vi "Entrenamiento Fuerza 2.vi"(8 "error in (no error)":errorcluster) -> (0 "error out":errorcluster, 3 "Message":string)   [LabVIEW 2014]
panel:
  out "Horizontal Graduated Bar":i16(slide) scale=0.0..100.0
  in  "Remove Button":bool
  in  "Add Button":bool
  out "Opcional %":string="0%"
  in  "Opcional Bool":bool
  out "Biceps %":string="0%"
  in  "Biceps Bool":bool
  out "Pectorales %":string="0%"
  in  "Pectorales Bool":bool
  out "Trapecio %":string="0%"
  in  "Trapecio Bool":bool
  out "Dorsales %":string="0%"
  in  "Dorsales Bool":bool
  out "Lumbares %":string="0%"
  in  "Lumbares Bool":bool
  out "Abdomen %":string="0%"
  in  "Abdomen Bool":bool
  out "Gluteos %":string="0%"
  in  "Gluteos Bool":bool
  out "Isquiotibiales %":string="0%"
  in  "Isquiotibiales Bool":bool
  in  "Stop":bool
  out "Cuadríceps %":string="0%"
  in  "Cuadriceps Bool":bool
  out "date/time string":string="22/08/2015 01:25:29 a. m."
  # "Entrenamiento de Fuerza"
  # "Presentación"
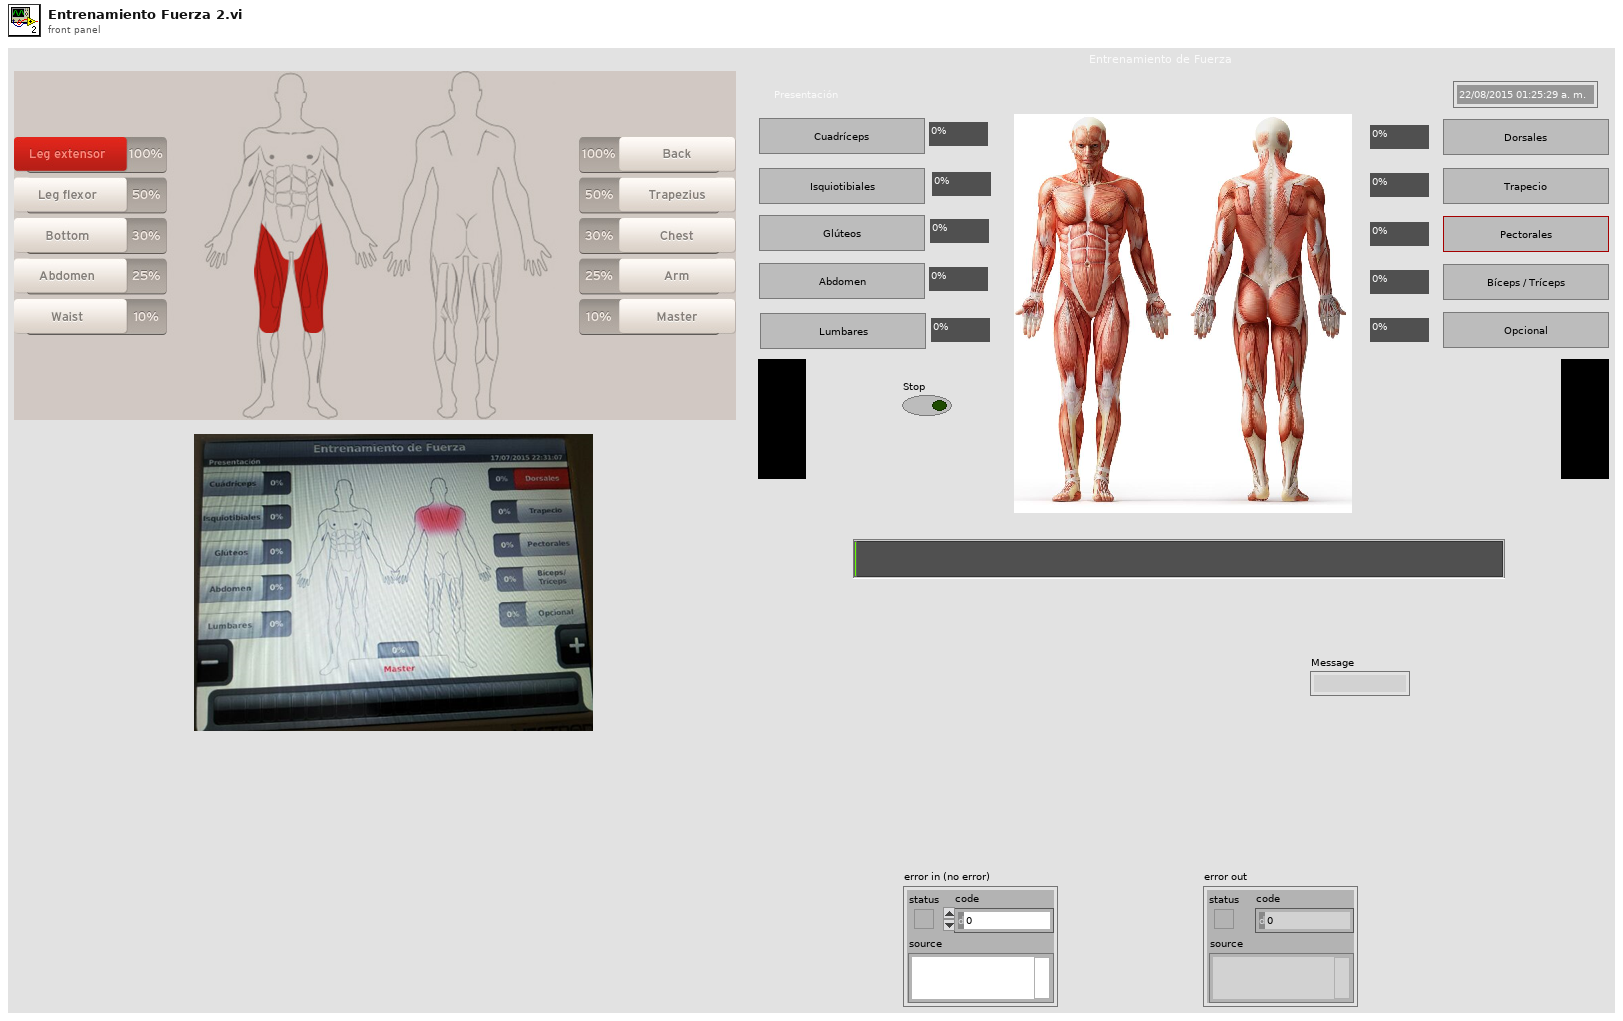
[diagram p1: front panel]
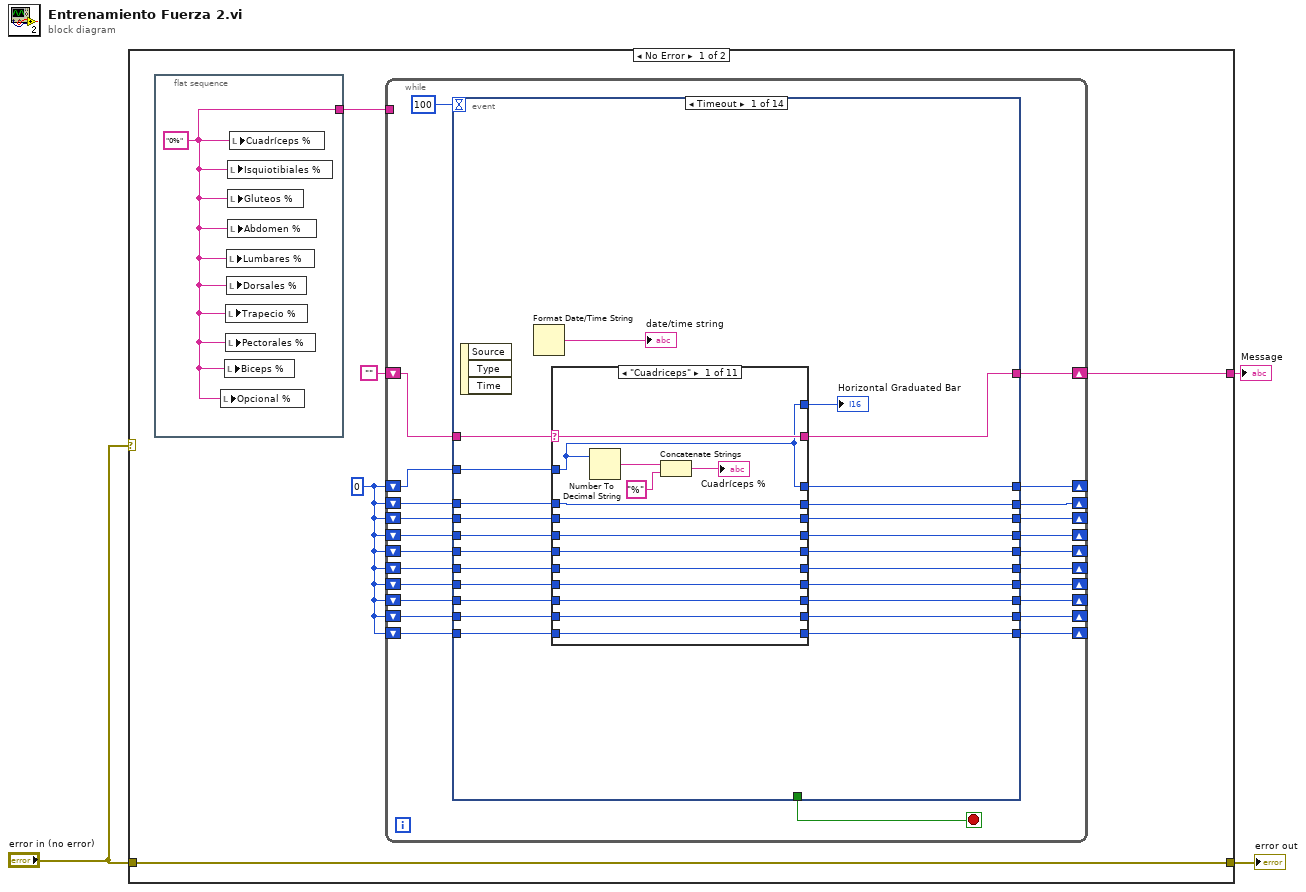
[diagram p0: block diagram]
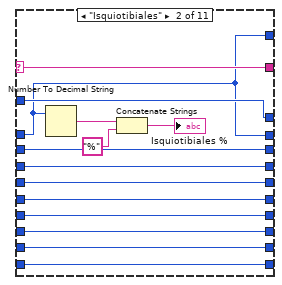
[diagram p2: hidden frame]
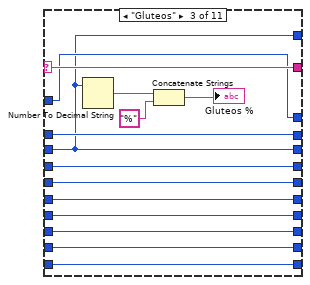
[diagram p3: hidden frame]
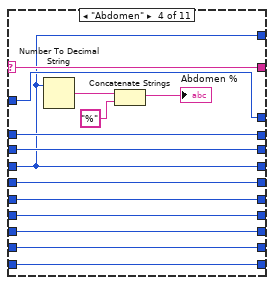
[diagram p4: hidden frame]
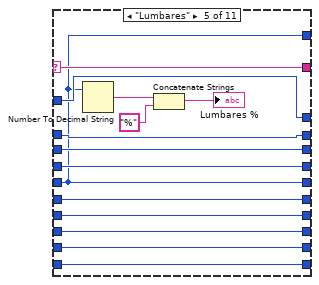
[diagram p5: hidden frame]
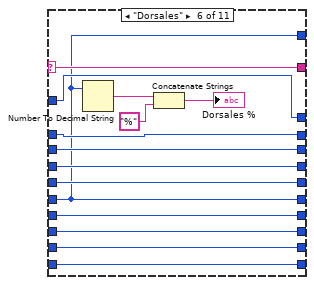
[diagram p6: hidden frame]
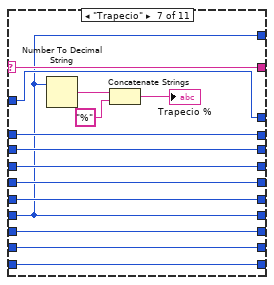
[diagram p7: hidden frame]
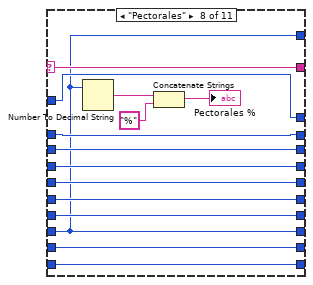
[diagram p8: hidden frame]
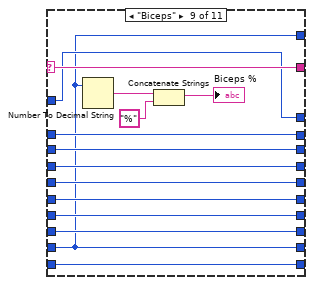
[diagram p9: hidden frame]
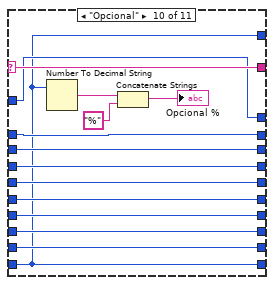
[diagram p10: hidden frame]
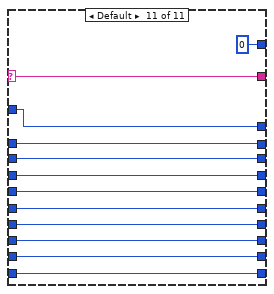
[diagram p11: hidden frame]
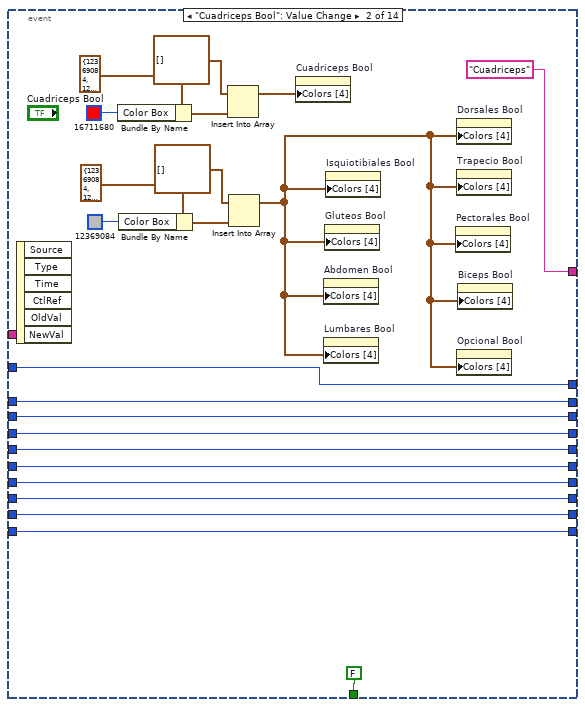
[diagram p12: hidden frame]
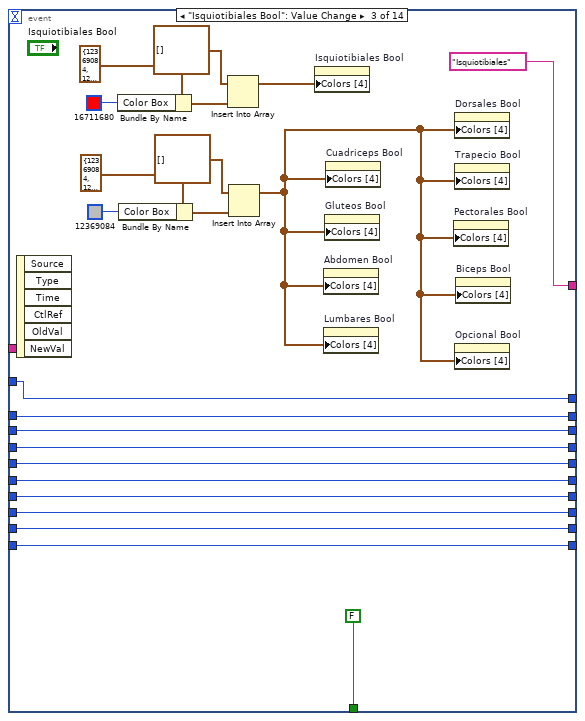
[diagram p13: hidden frame]
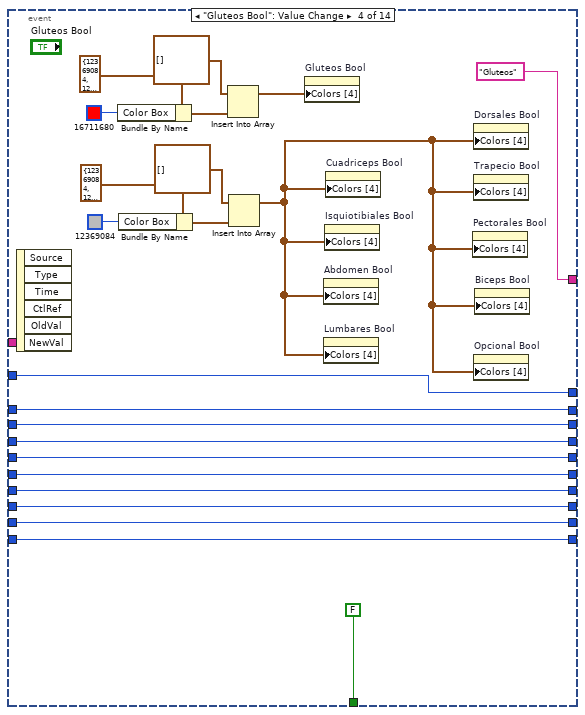
[diagram p14: hidden frame]
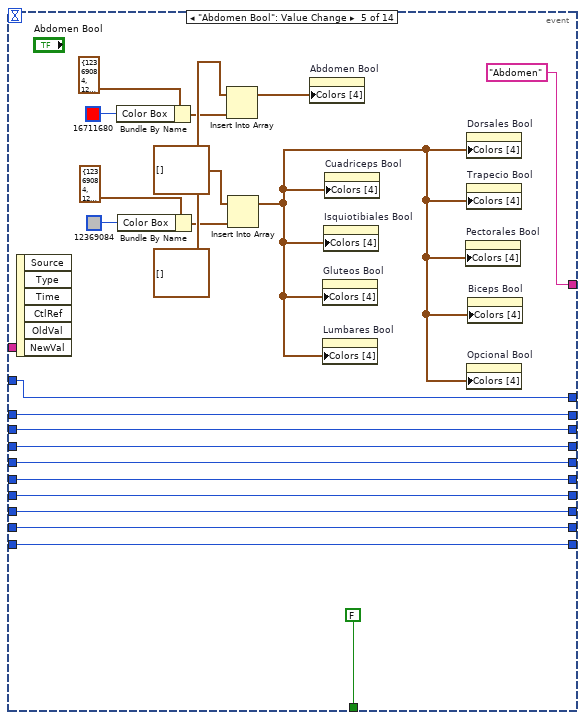
[diagram p15: hidden frame]
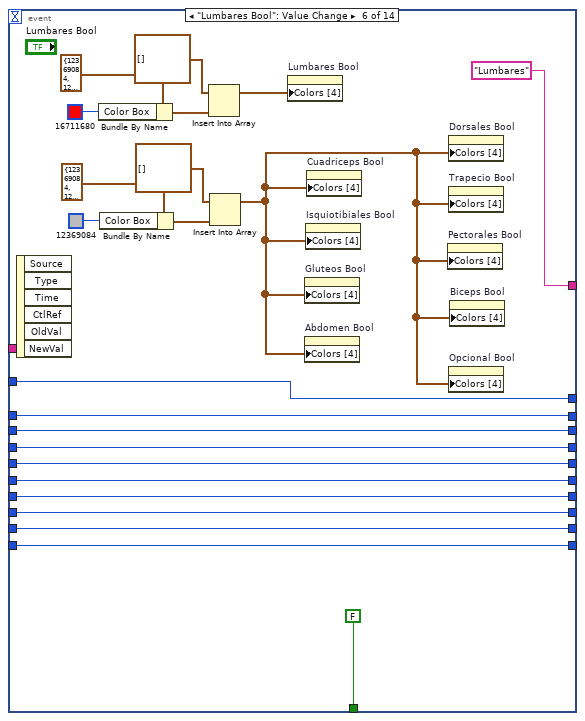
[diagram p16: hidden frame]
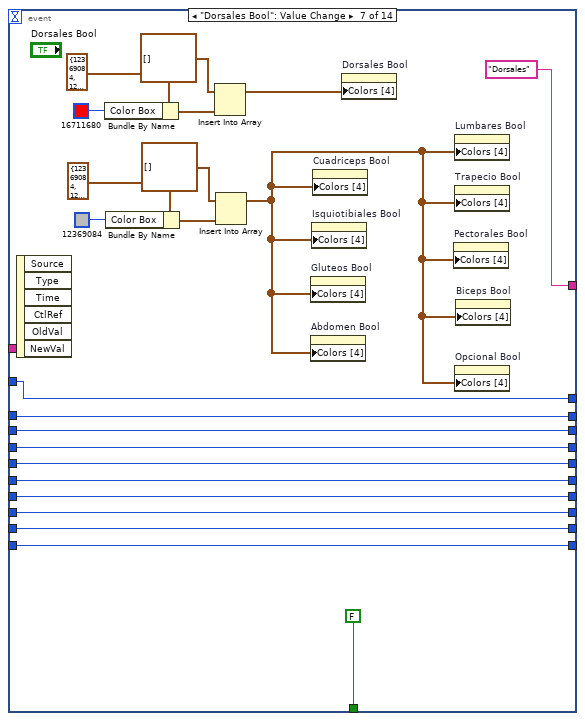
[diagram p17: hidden frame]
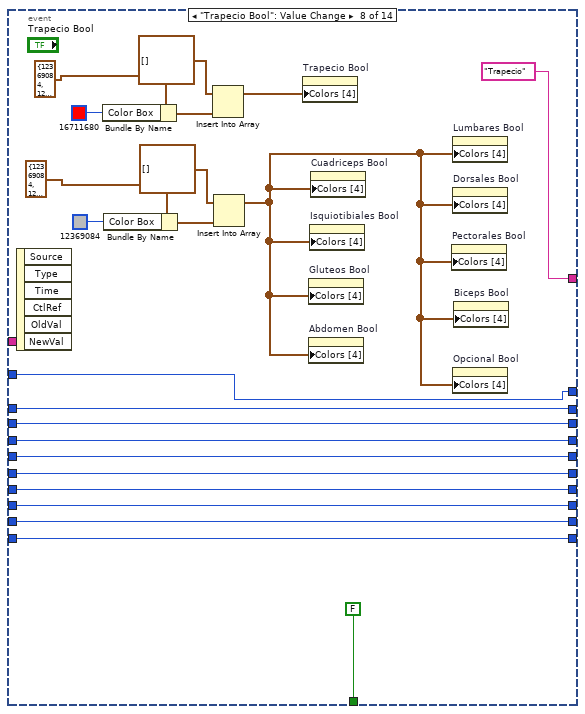
[diagram p18: hidden frame]
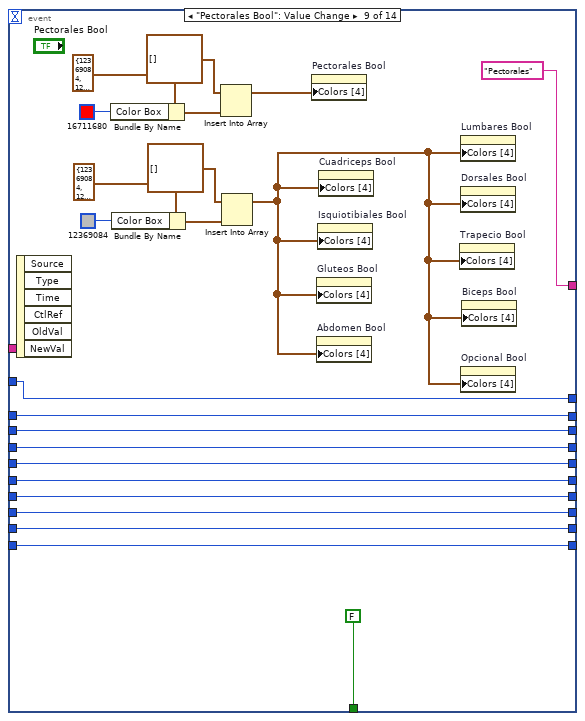
[diagram p19: hidden frame]
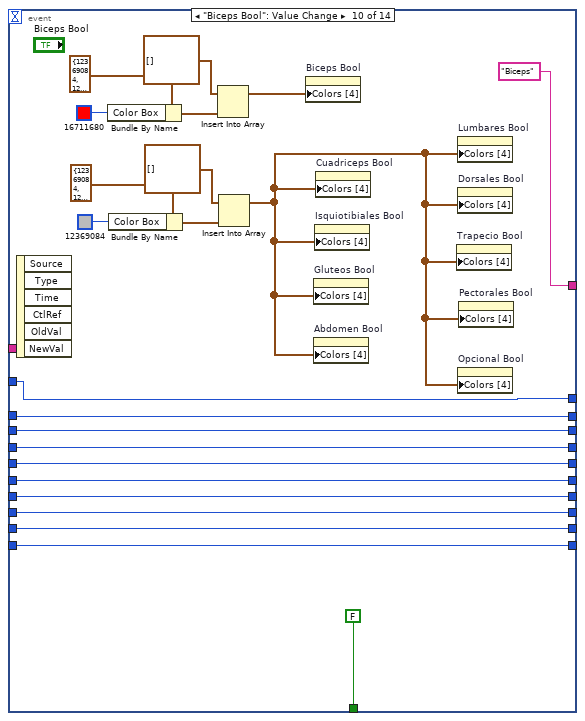
[diagram p20: hidden frame]
diagram:
  n1 = case shown="No Error" "error in (no error)" {
    tunnel: "error in (no error)" -> [w8 w815]
    tunnel: [w8 w815] -> w2
    tunnel: [w7 "Error" ("Message")] -> w1
    frame No Error {
      w5 = 0
      n2 = flat-sequence {
        tunnel: [w9] -> w4
        frame #0 {
          w9 = "0%" ("Cuadríceps %")
          n3 = local write "Opcional %"(w9) -> ()
          n4 = local write "Biceps %"(w9) -> ()
          n5 = local write "Trapecio %"(w9) -> ()
          n6 = local write "Pectorales %"(w9) -> ()
          n7 = local write "Lumbares %"(w9) -> ()
          n8 = local write "Dorsales %"(w9) -> ()
          n9 = local write "Isquiotibiales %"(w9) -> ()
          n10 = local write "Gluteos %"(w9) -> ()
          n11 = local write "Abdomen %"(w9) -> ()
          n12 = local write "Cuadríceps %"(w9) -> ()
        }
      }
      n13 = while {
        shift-right: [w31] -> w7
        shift-left: "" ("Message") -> [w30]
        shift-right: [w10] -> _
        shift-left: w5 -> [w29]
        shift-right: [w11] -> _
        shift-left: w5 -> [w28]
        shift-right: [w12] -> _
        shift-left: w5 -> [w27]
        shift-right: [w13] -> _
        shift-left: w5 -> [w26]
        shift-right: [w14] -> _
        shift-left: w5 -> [w25]
        shift-right: [w15] -> _
        shift-left: w5 -> [w24]
        shift-right: [w16] -> _
        shift-left: w5 -> [w23]
        shift-right: [w17] -> _
        shift-left: w5 -> [w22]
        shift-right: [w18] -> _
        shift-left: w5 -> [w21]
        shift-right: [w19] -> _
        shift-left: w5 -> [w20]
        tunnel: w4 -> [_]
        stop <- w33 stop-if-true
        n14 = event shown="[0] Timeout" {
          selector: _ -> [_ _ _ _ _ _ _ _ _ _ _ _ _ _]
          dyn-events: _ -> [_ _ _ _ _ _ _ _ _ _ _ _ _ _]
          timeout: 100 -> [_ _ _ _ _ _ _ _ _ _ _ _ _ _]
          tunnel: [_ FALSE FALSE FALSE FALSE FALSE FALSE FALSE FALSE FALSE FALSE _ _ "Stop"] -> w33
          tunnel: [w55 "Cuadriceps" ("Message") "Isquiotibiales" ("Message") "Gluteos" ("Message") "Abdomen" ("Message") "Lumbares" ("Message") "Dorsales" ("Message") "Trapecio" ("Message") "Pectorales" ("Message") "Biceps" ("Message") "Opcional" ("Message") w450 w651 w812] -> w31
          tunnel: w30 -> [w56 _ _ _ _ _ _ _ _ _ _ w450 w651 w812]
          tunnel: w29 -> [w54 w210 w241 w254 w276 w298 w329 w351 w364 w395 w417 w449 w650 w802]
          tunnel: w28 -> [w53 w211 w240 w255 w277 w299 w328 w350 w373 w394 w416 w440 w641 w803]
          tunnel: w27 -> [w52 w212 w239 w256 w278 w300 w327 w349 w372 w393 w415 w441 w642 w804]
          tunnel: w26 -> [w51 w213 w238 w257 w279 w301 w326 w348 w371 w392 w414 w442 w643 w805]
          tunnel: w25 -> [w50 w214 w237 w258 w280 w302 w325 w347 w370 w391 w413 w443 w644 w806]
          tunnel: w24 -> [w49 w215 w236 w259 w281 w303 w324 w346 w369 w390 w412 w444 w645 w807]
          tunnel: w23 -> [w48 w216 w235 w260 w282 w304 w323 w345 w368 w389 w411 w445 w646 w808]
          tunnel: w22 -> [w35 w217 w234 w261 w283 w305 w322 w344 w367 w388 w410 w446 w647 w809]
          tunnel: w21 -> [w47 w218 w233 w262 w284 w306 w321 w343 w366 w387 w409 w447 w648 w810]
          tunnel: w20 -> [w46 w219 w232 w263 w285 w307 w320 w342 w365 w386 w408 w448 w649 w811]
          tunnel: [w45 w219 w232 w263 w285 w307 w320 w342 w365 w386 w408 w431 w632 w811] -> w19
          tunnel: [w44 w218 w233 w262 w284 w306 w321 w343 w366 w387 w409 w432 w633 w810] -> w18
          tunnel: [w43 w217 w234 w261 w283 w305 w322 w344 w367 w388 w410 w433 w634 w809] -> w17
          tunnel: [w42 w216 w235 w260 w282 w304 w323 w345 w368 w389 w411 w434 w635 w808] -> w16
          tunnel: [w41 w215 w236 w259 w281 w303 w324 w346 w369 w390 w412 w435 w636 w807] -> w15
          tunnel: [w40 w214 w237 w258 w280 w302 w325 w347 w370 w391 w413 w436 w637 w806] -> w14
          tunnel: [w39 w213 w238 w257 w279 w301 w326 w348 w371 w392 w414 w437 w638 w805] -> w13
          tunnel: [w38 w212 w239 w256 w278 w300 w327 w349 w372 w393 w415 w438 w639 w804] -> w12
          tunnel: [w37 w211 w240 w255 w277 w299 w328 w350 w373 w394 w416 w439 w640 w803] -> w11
          tunnel: [w36 w210 w241 w254 w276 w298 w329 w351 w364 w395 w417 w430 w631 w802] -> w10
          event Timeout {
            n15 = event-data() -> ()  [unwired: 1 in, 3 out]
            n16 = Format Date/Time String() -> (date/time string=→"date/time string":string)  [unwired: 3 in]
            n17 = case shown="\"Cuadriceps\"" w56 {
              selector: w56 -> [w71 w85 w99 w113 w127 w141 w155 w169 w183 w197 w209]
              tunnel: [w71 w85 w99 w113 w127 w141 w155 w169 w183 w197 w209] -> w55
              tunnel: w54 -> [w58 w73 w87 w101 w115 w129 w143 w157 w171 w186 w208]
              tunnel: w53 -> [w59 w72 w88 w102 w116 w130 w144 w158 w172 w185 w207]
              tunnel: w52 -> [w60 w74 w86 w103 w117 w135 w145 w159 w173 w187 w206]
              tunnel: w51 -> [w61 w75 w89 w100 w118 w136 w146 w165 w174 w188 w205]
              tunnel: w50 -> [w62 w76 w90 w104 w114 w137 w147 w164 w175 w189 w204]
              tunnel: w49 -> [w63 w77 w91 w105 w123 w128 w148 w163 w176 w190 w203]
              tunnel: w48 -> [w64 w78 w92 w106 w122 w134 w142 w162 w177 w191 w202]
              tunnel: w47 -> [w66 w80 w94 w108 w120 w132 w151 w161 w170 w193 w200]
              tunnel: w46 -> [w67 w81 w95 w109 w119 w131 w149 w160 w179 w184 w199]
              tunnel: [w67 w81 w95 w109 w119 w131 w149 w160 w179 w184 w199] -> w45
              tunnel: [w66 w80 w94 w108 w120 w132 w151 w161 w170 w193 w200] -> w44
              tunnel: [w65 w79 w93 w107 w121 w133 w150 w156 w178 w192 w201] -> w43
              tunnel: [w64 w78 w92 w106 w122 w134 w142 w162 w177 w191 w202] -> w42
              tunnel: [w63 w77 w91 w105 w123 w128 w148 w163 w176 w190 w203] -> w41
              tunnel: [w62 w76 w90 w104 w114 w137 w147 w164 w175 w189 w204] -> w40
              tunnel: [w61 w75 w89 w100 w118 w136 w146 w165 w174 w188 w205] -> w39
              tunnel: [w60 w74 w86 w103 w117 w135 w145 w159 w173 w187 w206] -> w38
              tunnel: [w59 w72 w88 w102 w116 w130 w144 w158 w172 w185 w207] -> w37
              tunnel: [w58 w73 w87 w101 w115 w129 w143 w157 w171 w186 w208] -> w36
              tunnel: w35 -> [w65 w79 w93 w107 w121 w133 w150 w156 w178 w192 w201]
              tunnel: [w58 w72 w86 w100 w114 w128 w142 w156 w170 w184 0] -> w34
              frame "Cuadriceps" {
                n18 = Number To Decimal String(number=w58) -> (decimal integer string=w70:string)  [unwired: 1 in]
                n19 = Concatenate Strings(w70, "%" ("string")) -> (→"Cuadríceps %":string)
              }
              frame "Isquiotibiales" {
                n20 = Number To Decimal String(number=w72) -> (decimal integer string=w84:string)  [unwired: 1 in]
                n21 = Concatenate Strings(w84, "%" ("string")) -> (→"Isquiotibiales %":string)
              }
              frame "Gluteos" {
                n22 = Number To Decimal String(number=w86) -> (decimal integer string=w98:string)  [unwired: 1 in]
                n23 = Concatenate Strings(w98, "%" ("string")) -> (→"Gluteos %":string)
              }
              frame "Abdomen" {
                n24 = Number To Decimal String(number=w100) -> (decimal integer string=w112:string)  [unwired: 1 in]
                n25 = Concatenate Strings(w112, "%" ("string")) -> (→"Abdomen %":string)
              }
              frame "Lumbares" {
                n26 = Number To Decimal String(number=w114) -> (decimal integer string=w126:string)  [unwired: 1 in]
                n27 = Concatenate Strings(w126, "%" ("string")) -> (→"Lumbares %":string)
              }
              frame "Dorsales" {
                n28 = Number To Decimal String(number=w128) -> (decimal integer string=w140:string)  [unwired: 1 in]
                n29 = Concatenate Strings(w140, "%" ("string")) -> (→"Dorsales %":string)
              }
              frame "Trapecio" {
                n30 = Number To Decimal String(number=w142) -> (decimal integer string=w154:string)  [unwired: 1 in]
                n31 = Concatenate Strings(w154, "%" ("string")) -> (→"Trapecio %":string)
              }
              frame "Pectorales" {
                n32 = Number To Decimal String(number=w156) -> (decimal integer string=w168:string)  [unwired: 1 in]
                n33 = Concatenate Strings(w168, "%" ("string")) -> (→"Pectorales %":string)
              }
              frame "Biceps" {
                n34 = Number To Decimal String(number=w170) -> (decimal integer string=w182:string)  [unwired: 1 in]
                n35 = Concatenate Strings(w182, "%" ("string")) -> (→"Biceps %":string)
              }
              frame "Opcional" {
                n36 = Number To Decimal String(number=w184) -> (decimal integer string=w196:string)  [unwired: 1 in]
                n37 = Concatenate Strings(w196, "%" ("string")) -> (→"Opcional %":string)
              }
              frame Default {
              }
            }
            "Horizontal Graduated Bar" <- w34
          }
          event "Cuadriceps Bool": Value Change {
            n38 = event-data() -> ()  [unwired: 1 in, 6 out]
            n39 = Bundle By Name(cluster=cluster{"Color Box":u32, "Color Box 2":u32} {"Color Box"=12369084, "Color Box 2"=12369084}, "Color Box"=u32 16711680 ("Color Box 2")) -> (w228:cluster{"Color Box":u32, "Color Box 2":u32})
            n40 = Bundle By Name(cluster=cluster{"Color Box":u32, "Color Box 2":u32} {"Color Box"=12369084, "Color Box 2"=12369084}, "Color Box"=u32 12369084 ("Color Box 2")) -> (w223:cluster{"Color Box":u32, "Color Box 2":u32})
            n41 = Insert Into Array(array=cluster{u32, u32}[] [] ("Colors [4]"), new element=w228) -> (w227:cluster{u32, u32}[])  [unwired: 1 in]
            n42 = Insert Into Array(array=cluster{u32, u32}[] [] ("Colors [4]"), new element=w223) -> (w221:cluster{u32, u32}[])  [unwired: 1 in]
            n43 = property on="Cuadriceps Bool" class="Bool"("Colors [4]"=w227) -> ()  [unwired: 2 in, 2 out]
            n44 = property on="Abdomen Bool" class="Bool"("Colors [4]"=w221) -> ()  [unwired: 2 in, 2 out]
            n45 = property on="Lumbares Bool" class="Bool"("Colors [4]"=w221) -> ()  [unwired: 2 in, 2 out]
            n46 = property on="Gluteos Bool" class="Bool"("Colors [4]"=w221) -> ()  [unwired: 2 in, 2 out]
            n47 = property on="Isquiotibiales Bool" class="Bool"("Colors [4]"=w221) -> ()  [unwired: 2 in, 2 out]
            n48 = property on="Pectorales Bool" class="Bool"("Colors [4]"=w221) -> ()  [unwired: 2 in, 2 out]
            n49 = property on="Dorsales Bool" class="Bool"("Colors [4]"=w221) -> ()  [unwired: 2 in, 2 out]
            n50 = property on="Trapecio Bool" class="Bool"("Colors [4]"=w221) -> ()  [unwired: 2 in, 2 out]
            n51 = property on="Opcional Bool" class="Bool"("Colors [4]"=w221) -> ()  [unwired: 2 in, 2 out]
            n52 = property on="Biceps Bool" class="Bool"("Colors [4]"=w221) -> ()  [unwired: 2 in, 2 out]
          }
          event "Isquiotibiales Bool": Value Change {
            n53 = event-data() -> ()  [unwired: 1 in, 6 out]
            n54 = Bundle By Name(cluster=cluster{"Color Box":u32, "Color Box 2":u32} {"Color Box"=12369084, "Color Box 2"=12369084}, "Color Box"=u32 16711680 ("Color Box 2")) -> (w249:cluster{"Color Box":u32, "Color Box 2":u32})
            n55 = Bundle By Name(cluster=cluster{"Color Box":u32, "Color Box 2":u32} {"Color Box"=12369084, "Color Box 2"=12369084}, "Color Box"=u32 12369084 ("Color Box 2")) -> (w245:cluster{"Color Box":u32, "Color Box 2":u32})
            n56 = Insert Into Array(array=cluster{u32, u32}[] [] ("Colors [4]"), new element=w249) -> (w243:cluster{u32, u32}[])  [unwired: 1 in]
            n57 = Insert Into Array(array=cluster{u32, u32}[] [] ("Colors [4]"), new element=w245) -> (w242:cluster{u32, u32}[])  [unwired: 1 in]
            n58 = property on="Isquiotibiales Bool" class="Bool"("Colors [4]"=w243) -> ()  [unwired: 2 in, 2 out]
            n59 = property on="Abdomen Bool" class="Bool"("Colors [4]"=w242) -> ()  [unwired: 2 in, 2 out]
            n60 = property on="Lumbares Bool" class="Bool"("Colors [4]"=w242) -> ()  [unwired: 2 in, 2 out]
            n61 = property on="Gluteos Bool" class="Bool"("Colors [4]"=w242) -> ()  [unwired: 2 in, 2 out]
            n62 = property on="Cuadriceps Bool" class="Bool"("Colors [4]"=w242) -> ()  [unwired: 2 in, 2 out]
            n63 = property on="Pectorales Bool" class="Bool"("Colors [4]"=w242) -> ()  [unwired: 2 in, 2 out]
            n64 = property on="Dorsales Bool" class="Bool"("Colors [4]"=w242) -> ()  [unwired: 2 in, 2 out]
            n65 = property on="Trapecio Bool" class="Bool"("Colors [4]"=w242) -> ()  [unwired: 2 in, 2 out]
            n66 = property on="Opcional Bool" class="Bool"("Colors [4]"=w242) -> ()  [unwired: 2 in, 2 out]
            n67 = property on="Biceps Bool" class="Bool"("Colors [4]"=w242) -> ()  [unwired: 2 in, 2 out]
          }
          event "Gluteos Bool": Value Change {
            n68 = event-data() -> ()  [unwired: 1 in, 6 out]
            n69 = Bundle By Name(cluster=cluster{"Color Box":u32, "Color Box 2":u32} {"Color Box"=12369084, "Color Box 2"=12369084}, "Color Box"=u32 16711680 ("Color Box 2")) -> (w271:cluster{"Color Box":u32, "Color Box 2":u32})
            n70 = Bundle By Name(cluster=cluster{"Color Box":u32, "Color Box 2":u32} {"Color Box"=12369084, "Color Box 2"=12369084}, "Color Box"=u32 12369084 ("Color Box 2")) -> (w267:cluster{"Color Box":u32, "Color Box 2":u32})
            n71 = Insert Into Array(array=cluster{u32, u32}[] [] ("Colors [4]"), new element=w271) -> (w265:cluster{u32, u32}[])  [unwired: 1 in]
            n72 = Insert Into Array(array=cluster{u32, u32}[] [] ("Colors [4]"), new element=w267) -> (w264:cluster{u32, u32}[])  [unwired: 1 in]
            n73 = property on="Gluteos Bool" class="Bool"("Colors [4]"=w265) -> ()  [unwired: 2 in, 2 out]
            n74 = property on="Abdomen Bool" class="Bool"("Colors [4]"=w264) -> ()  [unwired: 2 in, 2 out]
            n75 = property on="Lumbares Bool" class="Bool"("Colors [4]"=w264) -> ()  [unwired: 2 in, 2 out]
            n76 = property on="Isquiotibiales Bool" class="Bool"("Colors [4]"=w264) -> ()  [unwired: 2 in, 2 out]
            n77 = property on="Cuadriceps Bool" class="Bool"("Colors [4]"=w264) -> ()  [unwired: 2 in, 2 out]
            n78 = property on="Pectorales Bool" class="Bool"("Colors [4]"=w264) -> ()  [unwired: 2 in, 2 out]
            n79 = property on="Dorsales Bool" class="Bool"("Colors [4]"=w264) -> ()  [unwired: 2 in, 2 out]
            n80 = property on="Trapecio Bool" class="Bool"("Colors [4]"=w264) -> ()  [unwired: 2 in, 2 out]
            n81 = property on="Opcional Bool" class="Bool"("Colors [4]"=w264) -> ()  [unwired: 2 in, 2 out]
            n82 = property on="Biceps Bool" class="Bool"("Colors [4]"=w264) -> ()  [unwired: 2 in, 2 out]
          }
          event "Abdomen Bool": Value Change {
            n83 = event-data() -> ()  [unwired: 1 in, 6 out]
            n84 = Bundle By Name(cluster=cluster{"Color Box":u32, "Color Box 2":u32} {"Color Box"=12369084, "Color Box 2"=12369084}, "Color Box"=u32 16711680 ("Color Box 2")) -> (w293:cluster{"Color Box":u32, "Color Box 2":u32})
            n85 = Bundle By Name(cluster=cluster{"Color Box":u32, "Color Box 2":u32} {"Color Box"=12369084, "Color Box 2"=12369084}, "Color Box"=u32 12369084 ("Color Box 2")) -> (w289:cluster{"Color Box":u32, "Color Box 2":u32})
            n86 = Insert Into Array(array=cluster{u32, u32}[] [] ("Colors [4]"), new element=w293) -> (w287:cluster{u32, u32}[])  [unwired: 1 in]
            n87 = Insert Into Array(array=cluster{u32, u32}[] [] ("Colors [4]"), new element=w289) -> (w286:cluster{u32, u32}[])  [unwired: 1 in]
            n88 = property on="Abdomen Bool" class="Bool"("Colors [4]"=w287) -> ()  [unwired: 2 in, 2 out]
            n89 = property on="Gluteos Bool" class="Bool"("Colors [4]"=w286) -> ()  [unwired: 2 in, 2 out]
            n90 = property on="Lumbares Bool" class="Bool"("Colors [4]"=w286) -> ()  [unwired: 2 in, 2 out]
            n91 = property on="Isquiotibiales Bool" class="Bool"("Colors [4]"=w286) -> ()  [unwired: 2 in, 2 out]
            n92 = property on="Cuadriceps Bool" class="Bool"("Colors [4]"=w286) -> ()  [unwired: 2 in, 2 out]
            n93 = property on="Pectorales Bool" class="Bool"("Colors [4]"=w286) -> ()  [unwired: 2 in, 2 out]
            n94 = property on="Dorsales Bool" class="Bool"("Colors [4]"=w286) -> ()  [unwired: 2 in, 2 out]
            n95 = property on="Trapecio Bool" class="Bool"("Colors [4]"=w286) -> ()  [unwired: 2 in, 2 out]
            n96 = property on="Opcional Bool" class="Bool"("Colors [4]"=w286) -> ()  [unwired: 2 in, 2 out]
            n97 = property on="Biceps Bool" class="Bool"("Colors [4]"=w286) -> ()  [unwired: 2 in, 2 out]
          }
          event "Lumbares Bool": Value Change {
            n98 = event-data() -> ()  [unwired: 1 in, 6 out]
            n99 = Bundle By Name(cluster=cluster{"Color Box":u32, "Color Box 2":u32} {"Color Box"=12369084, "Color Box 2"=12369084}, "Color Box"=u32 16711680 ("Color Box 2")) -> (w315:cluster{"Color Box":u32, "Color Box 2":u32})
            n100 = Bundle By Name(cluster=cluster{"Color Box":u32, "Color Box 2":u32} {"Color Box"=12369084, "Color Box 2"=12369084}, "Color Box"=u32 12369084 ("Color Box 2")) -> (w311:cluster{"Color Box":u32, "Color Box 2":u32})
            n101 = Insert Into Array(array=cluster{u32, u32}[] [] ("Colors [4]"), new element=w315) -> (w309:cluster{u32, u32}[])  [unwired: 1 in]
            n102 = Insert Into Array(array=cluster{u32, u32}[] [] ("Colors [4]"), new element=w311) -> (w308:cluster{u32, u32}[])  [unwired: 1 in]
            n103 = property on="Lumbares Bool" class="Bool"("Colors [4]"=w309) -> ()  [unwired: 2 in, 2 out]
            n104 = property on="Gluteos Bool" class="Bool"("Colors [4]"=w308) -> ()  [unwired: 2 in, 2 out]
            n105 = property on="Abdomen Bool" class="Bool"("Colors [4]"=w308) -> ()  [unwired: 2 in, 2 out]
            n106 = property on="Isquiotibiales Bool" class="Bool"("Colors [4]"=w308) -> ()  [unwired: 2 in, 2 out]
            n107 = property on="Cuadriceps Bool" class="Bool"("Colors [4]"=w308) -> ()  [unwired: 2 in, 2 out]
            n108 = property on="Pectorales Bool" class="Bool"("Colors [4]"=w308) -> ()  [unwired: 2 in, 2 out]
            n109 = property on="Dorsales Bool" class="Bool"("Colors [4]"=w308) -> ()  [unwired: 2 in, 2 out]
            n110 = property on="Trapecio Bool" class="Bool"("Colors [4]"=w308) -> ()  [unwired: 2 in, 2 out]
            n111 = property on="Opcional Bool" class="Bool"("Colors [4]"=w308) -> ()  [unwired: 2 in, 2 out]
            n112 = property on="Biceps Bool" class="Bool"("Colors [4]"=w308) -> ()  [unwired: 2 in, 2 out]
          }
          event "Dorsales Bool": Value Change {
            n113 = event-data() -> ()  [unwired: 1 in, 6 out]
            n114 = Bundle By Name(cluster=cluster{"Color Box":u32, "Color Box 2":u32} {"Color Box"=12369084, "Color Box 2"=12369084}, "Color Box"=u32 16711680 ("Color Box 2")) -> (w337:cluster{"Color Box":u32, "Color Box 2":u32})
            n115 = Bundle By Name(cluster=cluster{"Color Box":u32, "Color Box 2":u32} {"Color Box"=12369084, "Color Box 2"=12369084}, "Color Box"=u32 12369084 ("Color Box 2")) -> (w333:cluster{"Color Box":u32, "Color Box 2":u32})
            n116 = Insert Into Array(array=cluster{u32, u32}[] [] ("Colors [4]"), new element=w337) -> (w330:cluster{u32, u32}[])  [unwired: 1 in]
            n117 = Insert Into Array(array=cluster{u32, u32}[] [] ("Colors [4]"), new element=w333) -> (w331:cluster{u32, u32}[])  [unwired: 1 in]
            n118 = property on="Gluteos Bool" class="Bool"("Colors [4]"=w331) -> ()  [unwired: 2 in, 2 out]
            n119 = property on="Abdomen Bool" class="Bool"("Colors [4]"=w331) -> ()  [unwired: 2 in, 2 out]
            n120 = property on="Isquiotibiales Bool" class="Bool"("Colors [4]"=w331) -> ()  [unwired: 2 in, 2 out]
            n121 = property on="Cuadriceps Bool" class="Bool"("Colors [4]"=w331) -> ()  [unwired: 2 in, 2 out]
            n122 = property on="Dorsales Bool" class="Bool"("Colors [4]"=w330) -> ()  [unwired: 2 in, 2 out]
            n123 = property on="Pectorales Bool" class="Bool"("Colors [4]"=w331) -> ()  [unwired: 2 in, 2 out]
            n124 = property on="Lumbares Bool" class="Bool"("Colors [4]"=w331) -> ()  [unwired: 2 in, 2 out]
            n125 = property on="Trapecio Bool" class="Bool"("Colors [4]"=w331) -> ()  [unwired: 2 in, 2 out]
            n126 = property on="Opcional Bool" class="Bool"("Colors [4]"=w331) -> ()  [unwired: 2 in, 2 out]
            n127 = property on="Biceps Bool" class="Bool"("Colors [4]"=w331) -> ()  [unwired: 2 in, 2 out]
          }
          event "Trapecio Bool": Value Change {
            n128 = event-data() -> ()  [unwired: 1 in, 6 out]
            n129 = Bundle By Name(cluster=cluster{"Color Box":u32, "Color Box 2":u32} {"Color Box"=12369084, "Color Box 2"=12369084}, "Color Box"=u32 16711680 ("Color Box 2")) -> (w359:cluster{"Color Box":u32, "Color Box 2":u32})
            n130 = Bundle By Name(cluster=cluster{"Color Box":u32, "Color Box 2":u32} {"Color Box"=12369084, "Color Box 2"=12369084}, "Color Box"=u32 12369084 ("Color Box 2")) -> (w355:cluster{"Color Box":u32, "Color Box 2":u32})
            n131 = Insert Into Array(array=cluster{u32, u32}[] [] ("Colors [4]"), new element=w359) -> (w352:cluster{u32, u32}[])  [unwired: 1 in]
            n132 = Insert Into Array(array=cluster{u32, u32}[] [] ("Colors [4]"), new element=w355) -> (w353:cluster{u32, u32}[])  [unwired: 1 in]
            n133 = property on="Trapecio Bool" class="Bool"("Colors [4]"=w352) -> ()  [unwired: 2 in, 2 out]
            n134 = property on="Gluteos Bool" class="Bool"("Colors [4]"=w353) -> ()  [unwired: 2 in, 2 out]
            n135 = property on="Abdomen Bool" class="Bool"("Colors [4]"=w353) -> ()  [unwired: 2 in, 2 out]
            n136 = property on="Isquiotibiales Bool" class="Bool"("Colors [4]"=w353) -> ()  [unwired: 2 in, 2 out]
            n137 = property on="Cuadriceps Bool" class="Bool"("Colors [4]"=w353) -> ()  [unwired: 2 in, 2 out]
            n138 = property on="Pectorales Bool" class="Bool"("Colors [4]"=w353) -> ()  [unwired: 2 in, 2 out]
            n139 = property on="Lumbares Bool" class="Bool"("Colors [4]"=w353) -> ()  [unwired: 2 in, 2 out]
            n140 = property on="Dorsales Bool" class="Bool"("Colors [4]"=w353) -> ()  [unwired: 2 in, 2 out]
            n141 = property on="Opcional Bool" class="Bool"("Colors [4]"=w353) -> ()  [unwired: 2 in, 2 out]
            n142 = property on="Biceps Bool" class="Bool"("Colors [4]"=w353) -> ()  [unwired: 2 in, 2 out]
          }
          event "Pectorales Bool": Value Change {
            n143 = event-data() -> ()  [unwired: 1 in, 6 out]
            n144 = Bundle By Name(cluster=cluster{"Color Box":u32, "Color Box 2":u32} {"Color Box"=12369084, "Color Box 2"=12369084}, "Color Box"=u32 16711680 ("Color Box 2")) -> (w381:cluster{"Color Box":u32, "Color Box 2":u32})
            n145 = Bundle By Name(cluster=cluster{"Color Box":u32, "Color Box 2":u32} {"Color Box"=12369084, "Color Box 2"=12369084}, "Color Box"=u32 12369084 ("Color Box 2")) -> (w377:cluster{"Color Box":u32, "Color Box 2":u32})
            n146 = Insert Into Array(array=cluster{u32, u32}[] [] ("Colors [4]"), new element=w381) -> (w374:cluster{u32, u32}[])  [unwired: 1 in]
            n147 = Insert Into Array(array=cluster{u32, u32}[] [] ("Colors [4]"), new element=w377) -> (w375:cluster{u32, u32}[])  [unwired: 1 in]
            n148 = property on="Pectorales Bool" class="Bool"("Colors [4]"=w374) -> ()  [unwired: 2 in, 2 out]
            n149 = property on="Gluteos Bool" class="Bool"("Colors [4]"=w375) -> ()  [unwired: 2 in, 2 out]
            n150 = property on="Abdomen Bool" class="Bool"("Colors [4]"=w375) -> ()  [unwired: 2 in, 2 out]
            n151 = property on="Isquiotibiales Bool" class="Bool"("Colors [4]"=w375) -> ()  [unwired: 2 in, 2 out]
            n152 = property on="Cuadriceps Bool" class="Bool"("Colors [4]"=w375) -> ()  [unwired: 2 in, 2 out]
            n153 = property on="Trapecio Bool" class="Bool"("Colors [4]"=w375) -> ()  [unwired: 2 in, 2 out]
            n154 = property on="Lumbares Bool" class="Bool"("Colors [4]"=w375) -> ()  [unwired: 2 in, 2 out]
            n155 = property on="Dorsales Bool" class="Bool"("Colors [4]"=w375) -> ()  [unwired: 2 in, 2 out]
            n156 = property on="Opcional Bool" class="Bool"("Colors [4]"=w375) -> ()  [unwired: 2 in, 2 out]
            n157 = property on="Biceps Bool" class="Bool"("Colors [4]"=w375) -> ()  [unwired: 2 in, 2 out]
          }
          event "Biceps Bool": Value Change {
            n158 = event-data() -> ()  [unwired: 1 in, 6 out]
            n159 = Bundle By Name(cluster=cluster{"Color Box":u32, "Color Box 2":u32} {"Color Box"=12369084, "Color Box 2"=12369084}, "Color Box"=u32 16711680 ("Color Box 2")) -> (w404:cluster{"Color Box":u32, "Color Box 2":u32})
            n160 = Bundle By Name(cluster=cluster{"Color Box":u32, "Color Box 2":u32} {"Color Box"=12369084, "Color Box 2"=12369084}, "Color Box"=u32 12369084 ("Color Box 2")) -> (w400:cluster{"Color Box":u32, "Color Box 2":u32})
            n161 = Insert Into Array(array=cluster{u32, u32}[] [] ("Colors [4]"), new element=w404) -> (w397:cluster{u32, u32}[])  [unwired: 1 in]
            n162 = Insert Into Array(array=cluster{u32, u32}[] [] ("Colors [4]"), new element=w400) -> (w398:cluster{u32, u32}[])  [unwired: 1 in]
            n163 = property on="Biceps Bool" class="Bool"("Colors [4]"=w397) -> ()  [unwired: 2 in, 2 out]
            n164 = property on="Gluteos Bool" class="Bool"("Colors [4]"=w398) -> ()  [unwired: 2 in, 2 out]
            n165 = property on="Abdomen Bool" class="Bool"("Colors [4]"=w398) -> ()  [unwired: 2 in, 2 out]
            n166 = property on="Isquiotibiales Bool" class="Bool"("Colors [4]"=w398) -> ()  [unwired: 2 in, 2 out]
            n167 = property on="Cuadriceps Bool" class="Bool"("Colors [4]"=w398) -> ()  [unwired: 2 in, 2 out]
            n168 = property on="Trapecio Bool" class="Bool"("Colors [4]"=w398) -> ()  [unwired: 2 in, 2 out]
            n169 = property on="Lumbares Bool" class="Bool"("Colors [4]"=w398) -> ()  [unwired: 2 in, 2 out]
            n170 = property on="Dorsales Bool" class="Bool"("Colors [4]"=w398) -> ()  [unwired: 2 in, 2 out]
            n171 = property on="Opcional Bool" class="Bool"("Colors [4]"=w398) -> ()  [unwired: 2 in, 2 out]
            n172 = property on="Pectorales Bool" class="Bool"("Colors [4]"=w398) -> ()  [unwired: 2 in, 2 out]
          }
          event "Opcional Bool": Value Change {
            n173 = event-data() -> ()  [unwired: 1 in, 6 out]
            n174 = Bundle By Name(cluster=cluster{"Color Box":u32, "Color Box 2":u32} {"Color Box"=12369084, "Color Box 2"=12369084}, "Color Box"=u32 16711680 ("Color Box 2")) -> (w425:cluster{"Color Box":u32, "Color Box 2":u32})
            n175 = Bundle By Name(cluster=cluster{"Color Box":u32, "Color Box 2":u32} {"Color Box"=12369084, "Color Box 2"=12369084}, "Color Box"=u32 12369084 ("Color Box 2")) -> (w421:cluster{"Color Box":u32, "Color Box 2":u32})
            n176 = Insert Into Array(array=cluster{u32, u32}[] [] ("Colors [4]"), new element=w425) -> (w418:cluster{u32, u32}[])  [unwired: 1 in]
            n177 = Insert Into Array(array=cluster{u32, u32}[] [] ("Colors [4]"), new element=w421) -> (w419:cluster{u32, u32}[])  [unwired: 1 in]
            n178 = property on="Opcional Bool" class="Bool"("Colors [4]"=w418) -> ()  [unwired: 2 in, 2 out]
            n179 = property on="Gluteos Bool" class="Bool"("Colors [4]"=w419) -> ()  [unwired: 2 in, 2 out]
            n180 = property on="Abdomen Bool" class="Bool"("Colors [4]"=w419) -> ()  [unwired: 2 in, 2 out]
            n181 = property on="Isquiotibiales Bool" class="Bool"("Colors [4]"=w419) -> ()  [unwired: 2 in, 2 out]
            n182 = property on="Cuadriceps Bool" class="Bool"("Colors [4]"=w419) -> ()  [unwired: 2 in, 2 out]
            n183 = property on="Trapecio Bool" class="Bool"("Colors [4]"=w419) -> ()  [unwired: 2 in, 2 out]
            n184 = property on="Lumbares Bool" class="Bool"("Colors [4]"=w419) -> ()  [unwired: 2 in, 2 out]
            n185 = property on="Dorsales Bool" class="Bool"("Colors [4]"=w419) -> ()  [unwired: 2 in, 2 out]
            n186 = property on="Biceps Bool" class="Bool"("Colors [4]"=w419) -> ()  [unwired: 2 in, 2 out]
            n187 = property on="Pectorales Bool" class="Bool"("Colors [4]"=w419) -> ()  [unwired: 2 in, 2 out]
          }
          event "Add Button": Value Change {
            n188 = event-data() -> ()  [unwired: 1 in, 6 out]
            n189 = case shown="\"Cuadriceps\"" w450 {
              tunnel: w449 -> [w461 w470 w488 w506 w524 w542 w560 w578 w596 w614 w630]
              tunnel: w448 -> [w460 w478 w495 w512 w529 w546 w563 w580 w597 w605 w621]
              tunnel: w447 -> [w459 w477 w494 w511 w528 w545 w562 w579 w587 w606 w622]
              tunnel: w446 -> [w458 w476 w493 w510 w527 w544 w561 w572 w589 w607 w623]
              tunnel: w445 -> [w457 w475 w492 w509 w526 w543 w554 w571 w590 w608 w624]
              tunnel: w444 -> [w456 w474 w491 w508 w525 w536 w555 w573 w591 w609 w625]
              tunnel: w443 -> [w455 w473 w490 w507 w520 w538 w556 w574 w592 w610 w626]
              tunnel: w442 -> [w454 w472 w489 w503 w521 w539 w557 w575 w593 w611 w627]
              tunnel: w441 -> [w453 w471 w486 w504 w522 w540 w558 w576 w594 w612 w628]
              tunnel: w440 -> [w452 w469 w487 w505 w523 w541 w559 w577 w595 w613 w629]
              tunnel: [w460 w478 w495 w512 w529 w546 w563 w580 w597 w604 w621] -> w431
              tunnel: [w459 w477 w494 w511 w528 w545 w562 w579 w588 w606 w622] -> w432
              tunnel: [w458 w476 w493 w510 w527 w544 w561 w570 w589 w607 w623] -> w433
              tunnel: [w457 w475 w492 w509 w526 w543 w553 w571 w590 w608 w624] -> w434
              tunnel: [w456 w474 w491 w508 w525 w537 w555 w573 w591 w609 w625] -> w435
              tunnel: [w455 w473 w490 w507 w519 w538 w556 w574 w592 w610 w626] -> w436
              tunnel: [w454 w472 w489 w502 w521 w539 w557 w575 w593 w611 w627] -> w437
              tunnel: [w453 w471 w485 w504 w522 w540 w558 w576 w594 w612 w628] -> w438
              tunnel: [w452 w468 w487 w505 w523 w541 w559 w577 w595 w613 w629] -> w439
              tunnel: [w451 w470 w488 w506 w524 w542 w560 w578 w596 w614 w630] -> w430
              frame "Cuadriceps" {
                n190 = Greater Or Equal To 0?(x=w461) -> (x >= 0?=w465:bool)
                n191 = Less Or Equal?(x=w461, y=100) -> (x <= y?=w463:bool)
                n192 = Add(x=w461, y=5) -> (x+y=w467:i32)
                n193 = And(x=w465, y=w463) -> (x .and. y?=w464:bool)
                n194 = Select(t=w467, s=w464, f=w461) -> (s? t:f=w451:i32)
              }
              frame "Isquiotibiales" {
                n195 = Greater Or Equal To 0?(x=w469) -> (x >= 0?=w482:bool)
                n196 = Less Or Equal?(x=w469, y=100) -> (x <= y?=w480:bool)
                n197 = Add(x=w469, y=5) -> (x+y=w484:i32)
                n198 = And(x=w482, y=w480) -> (x .and. y?=w481:bool)
                n199 = Select(t=w484, s=w481, f=w469) -> (s? t:f=w468:i32)
              }
              frame "Gluteos" {
                n200 = Greater Or Equal To 0?(x=w486) -> (x >= 0?=w499:bool)
                n201 = Less Or Equal?(x=w486, y=100) -> (x <= y?=w497:bool)
                n202 = Add(x=w486, y=5) -> (x+y=w501:i32)
                n203 = And(x=w499, y=w497) -> (x .and. y?=w498:bool)
                n204 = Select(t=w501, s=w498, f=w486) -> (s? t:f=w485:i32)
              }
              frame "Abdomen" {
                n205 = Greater Or Equal To 0?(x=w503) -> (x >= 0?=w516:bool)
                n206 = Less Or Equal?(x=w503, y=100) -> (x <= y?=w514:bool)
                n207 = Add(x=w503, y=5) -> (x+y=w518:i32)
                n208 = And(x=w516, y=w514) -> (x .and. y?=w515:bool)
                n209 = Select(t=w518, s=w515, f=w503) -> (s? t:f=w502:i32)
              }
              frame "Lumbares" {
                n210 = Greater Or Equal To 0?(x=w520) -> (x >= 0?=w533:bool)
                n211 = Less Or Equal?(x=w520, y=100) -> (x <= y?=w531:bool)
                n212 = Add(x=w520, y=5) -> (x+y=w535:i32)
                n213 = And(x=w533, y=w531) -> (x .and. y?=w532:bool)
                n214 = Select(t=w535, s=w532, f=w520) -> (s? t:f=w519:i32)
              }
              frame "Dorsales" {
                n215 = Greater Or Equal To 0?(x=w536) -> (x >= 0?=w550:bool)
                n216 = Less Or Equal?(x=w536, y=100) -> (x <= y?=w548:bool)
                n217 = Add(x=w536, y=5) -> (x+y=w552:i32)
                n218 = And(x=w550, y=w548) -> (x .and. y?=w549:bool)
                n219 = Select(t=w552, s=w549, f=w536) -> (s? t:f=w537:i32)
              }
              frame "Trapecio" {
                n220 = Greater Or Equal To 0?(x=w554) -> (x >= 0?=w567:bool)
                n221 = Less Or Equal?(x=w554, y=100) -> (x <= y?=w565:bool)
                n222 = Add(x=w554, y=5) -> (x+y=w569:i32)
                n223 = And(x=w567, y=w565) -> (x .and. y?=w566:bool)
                n224 = Select(t=w569, s=w566, f=w554) -> (s? t:f=w553:i32)
              }
              frame "Pectorales" {
                n225 = Greater Or Equal To 0?(x=w572) -> (x >= 0?=w584:bool)
                n226 = Less Or Equal?(x=w572, y=100) -> (x <= y?=w582:bool)
                n227 = Add(x=w572, y=5) -> (x+y=w586:i32)
                n228 = And(x=w584, y=w582) -> (x .and. y?=w583:bool)
                n229 = Select(t=w586, s=w583, f=w572) -> (s? t:f=w570:i32)
              }
              frame "Biceps" {
                n230 = Greater Or Equal To 0?(x=w587) -> (x >= 0?=w601:bool)
                n231 = Less Or Equal?(x=w587, y=100) -> (x <= y?=w599:bool)
                n232 = Add(x=w587, y=5) -> (x+y=w603:i32)
                n233 = And(x=w601, y=w599) -> (x .and. y?=w600:bool)
                n234 = Select(t=w603, s=w600, f=w587) -> (s? t:f=w588:i32)
              }
              frame "Opcional" {
                n235 = Greater Or Equal To 0?(x=w605) -> (x >= 0?=w618:bool)
                n236 = Less Or Equal?(x=w605, y=100) -> (x <= y?=w616:bool)
                n237 = Add(x=w605, y=5) -> (x+y=w620:i32)
                n238 = And(x=w618, y=w616) -> (x .and. y?=w617:bool)
                n239 = Select(t=w620, s=w617, f=w605) -> (s? t:f=w604:i32)
              }
              frame Default {
              }
            }
          }
          event "Remove Button": Value Change {
            n240 = event-data() -> ()  [unwired: 1 in, 6 out]
            n241 = case shown="\"Cuadriceps\"" w651 {
              tunnel: w650 -> [w652 w671 w686 w701 w716 w731 w746 w761 w776 w791 w801]
              tunnel: w649 -> [w665 w679 w693 w707 w721 w735 w749 w763 w777 w778 w792]
              tunnel: w648 -> [w664 w678 w692 w706 w720 w734 w748 w762 w764 w783 w793]
              tunnel: w647 -> [w663 w677 w691 w705 w719 w733 w747 w750 w769 w784 w794]
              tunnel: w646 -> [w662 w676 w690 w704 w718 w732 w737 w755 w770 w785 w795]
              tunnel: w645 -> [w661 w675 w689 w703 w717 w722 w741 w756 w771 w786 w796]
              tunnel: w644 -> [w660 w674 w688 w702 w708 w727 w742 w757 w772 w787 w797]
              tunnel: w643 -> [w659 w673 w687 w694 w713 w728 w743 w758 w773 w788 w798]
              tunnel: w642 -> [w658 w672 w680 w699 w714 w729 w744 w759 w774 w789 w799]
              tunnel: w641 -> [w657 w666 w685 w700 w715 w730 w745 w760 w775 w790 w800]
              tunnel: [w665 w679 w693 w707 w721 w735 w749 w763 w777 w779 w792] -> w632
              tunnel: [w664 w678 w692 w706 w720 w734 w748 w762 w765 w783 w793] -> w633
              tunnel: [w663 w677 w691 w705 w719 w733 w747 w751 w769 w784 w794] -> w634
              tunnel: [w662 w676 w690 w704 w718 w732 w736 w755 w770 w785 w795] -> w635
              tunnel: [w661 w675 w689 w703 w717 w723 w741 w756 w771 w786 w796] -> w636
              tunnel: [w660 w674 w688 w702 w709 w727 w742 w757 w772 w787 w797] -> w637
              tunnel: [w659 w673 w687 w695 w713 w728 w743 w758 w773 w788 w798] -> w638
              tunnel: [w658 w672 w681 w699 w714 w729 w744 w759 w774 w789 w799] -> w639
              tunnel: [w657 w667 w685 w700 w715 w730 w745 w760 w775 w790 w800] -> w640
              tunnel: [w653 w671 w686 w701 w716 w731 w746 w761 w776 w791 w801] -> w631
              frame "Cuadriceps" {
                n242 = Greater Than 0?(x=w652) -> (x > 0?=w656:bool)
                n243 = Subtract(x=w652, y=5) -> (x-y=w655:i32)
                n244 = Select(t=w655, s=w656, f=w652) -> (s? t:f=w653:i32)
              }
              frame "Isquiotibiales" {
                n245 = Greater Than 0?(x=w666) -> (x > 0?=w670:bool)
                n246 = Subtract(x=w666, y=5) -> (x-y=w669:i32)
                n247 = Select(t=w669, s=w670, f=w666) -> (s? t:f=w667:i32)
              }
              frame "Gluteos" {
                n248 = Greater Than 0?(x=w680) -> (x > 0?=w684:bool)
                n249 = Subtract(x=w680, y=5) -> (x-y=w683:i32)
                n250 = Select(t=w683, s=w684, f=w680) -> (s? t:f=w681:i32)
              }
              frame "Abdomen" {
                n251 = Greater Than 0?(x=w694) -> (x > 0?=w698:bool)
                n252 = Subtract(x=w694, y=5) -> (x-y=w697:i32)
                n253 = Select(t=w697, s=w698, f=w694) -> (s? t:f=w695:i32)
              }
              frame "Lumbares" {
                n254 = Greater Than 0?(x=w708) -> (x > 0?=w712:bool)
                n255 = Subtract(x=w708, y=5) -> (x-y=w711:i32)
                n256 = Select(t=w711, s=w712, f=w708) -> (s? t:f=w709:i32)
              }
              frame "Dorsales" {
                n257 = Greater Than 0?(x=w722) -> (x > 0?=w726:bool)
                n258 = Subtract(x=w722, y=5) -> (x-y=w725:i32)
                n259 = Select(t=w725, s=w726, f=w722) -> (s? t:f=w723:i32)
              }
              frame "Trapecio" {
                n260 = Greater Than 0?(x=w737) -> (x > 0?=w740:bool)
                n261 = Subtract(x=w737, y=5) -> (x-y=w739:i32)
                n262 = Select(t=w739, s=w740, f=w737) -> (s? t:f=w736:i32)
              }
              frame "Pectorales" {
                n263 = Greater Than 0?(x=w750) -> (x > 0?=w754:bool)
                n264 = Subtract(x=w750, y=5) -> (x-y=w753:i32)
                n265 = Select(t=w753, s=w754, f=w750) -> (s? t:f=w751:i32)
              }
              frame "Biceps" {
                n266 = Greater Than 0?(x=w764) -> (x > 0?=w768:bool)
                n267 = Subtract(x=w764, y=5) -> (x-y=w767:i32)
                n268 = Select(t=w767, s=w768, f=w764) -> (s? t:f=w765:i32)
              }
              frame "Opcional" {
                n269 = Greater Than 0?(x=w778) -> (x > 0?=w782:bool)
                n270 = Subtract(x=w778, y=5) -> (x-y=w781:i32)
                n271 = Select(t=w781, s=w782, f=w778) -> (s? t:f=w779:i32)
              }
              frame Default {
              }
            }
          }
          event "Stop": Value Change {
            n272 = event-data() -> ()  [unwired: 1 in, 6 out]
          }
        }
      }
    }
    frame Error {
    }
  }
  "error out" <- w2
  "Message" <- w1
